vi "GV FIFOOUT gate.vi"() -> ()   [LabVIEW 2017]
panel:
  out "FIFOOUT gate":bool
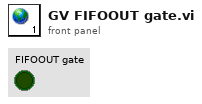
[diagram p1: front panel]
diagram:
